vi "CylFGV.vi"(9 "Action":T3(ring), 10 "Index":i8, 11 "SEQ in":T1 {"Delay Time" format="%.3f"}) -> (1 "SEQ Pool":T2(array[cluster]) {"Delay Time" format="%.3f"}, 2 "Size":i8, 3 "SEQ out":T1 {"Delay Time" format="%.3f"})   [LabVIEW 2012, in "StimulCtrls.lvlib"]
uses:
  StimulCtrls.lvlib
  Sequence.lvclass
panel:
  # "Functional global variable used to store SEQ pool"
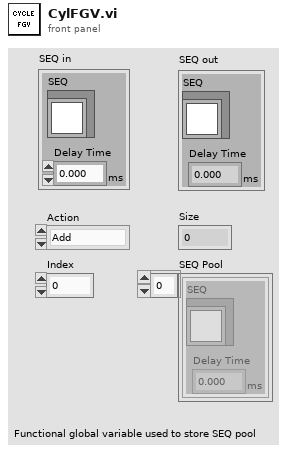
[diagram p1: front panel]
types:
  T1 = cluster{"SEQ":refnum<class "Sequence.lvclass">, "Delay Time":dbl[unit]}
  T2 = cluster{"SEQ":refnum<class "Sequence.lvclass">, "Delay Time":dbl[unit]}[]
  T3 = enum16{"Add", "New", "Del", "Update", "Get", "Initial", "GetSize"}
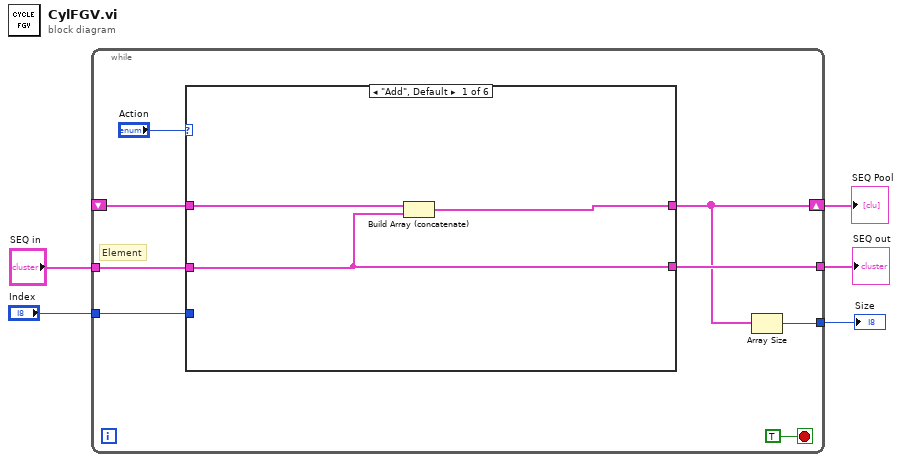
[diagram p0: block diagram]
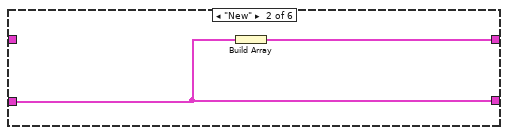
[diagram p2: hidden frame]
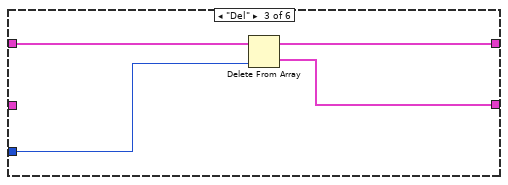
[diagram p3: hidden frame]
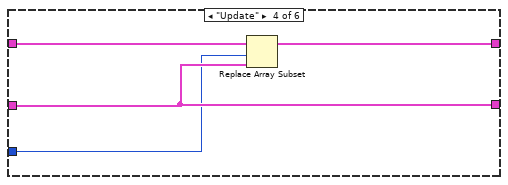
[diagram p4: hidden frame]
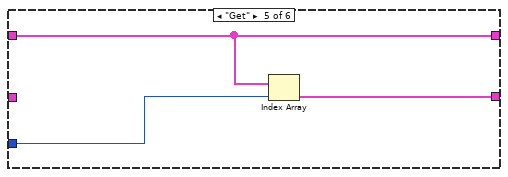
[diagram p5: hidden frame]
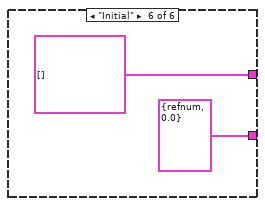
[diagram p6: hidden frame]
diagram:
  n1 = while {
    tunnel: "SEQ in" -> [w11]
    shift-right: [w7] -> w4
    shift-left: _ -> [w10]
    tunnel: [w9] -> w1
    tunnel: [w8] -> w5
    tunnel: "Index" -> [w6]
    stop <- TRUE stop-if-true
    # "Element"
    n2 = case shown="\"Add\", Default" "Action" {
      tunnel: w11 -> [w14 w17 _ w24 _ _]
      tunnel: w10 -> [w16 _ w22 w26 w29 _]
      tunnel: [w15 w18 w20 w25 w29 T2 []] -> w7
      tunnel: w6 -> [_ _ w21 w23 w28 _]
      tunnel: [w14 w17 w19 w24 w27 T1 {"SEQ"=refnum, "Delay Time"=0.0} ("SEQ in")] -> w9
      frame "Add", Default {
        n3 = Build Array (concatenate)(w16, w14) -> (w15:T2)
      }
      frame "New" {
        n4 = Build Array(w17) -> (w18:T2)
      }
      frame "Del" {
        n5 = Delete From Array(array=w22, index=w21) -> (deleted portion=w19:T1, array with subset deleted=w20:T2)  [unwired: 1 in]
      }
      frame "Update" {
        n6 = Replace Array Subset(array=w26, new element=w24, index=w23) -> (w25:T2)
      }
      frame "Get" {
        n7 = Index Array(array=w29, index=w28) -> (element=w27:T1)
      }
      frame "Initial" {
      }
    }
    n8 = Array Size(array=w7) -> (size(s)=w8:i32)
  }
  "Size" <- w5
  "SEQ Pool" <- w4
  "SEQ out" <- w1
